vi "Voltage to temperature.vi"(8 "error in (no error)":errorcluster, 11 "Input Voltage (V)":dbl) -> (0 "error out":errorcluster, 3 "Temperature (C)":dbl)   [LabVIEW 2014]
doc: "Converts the input voltage to illuminance result."
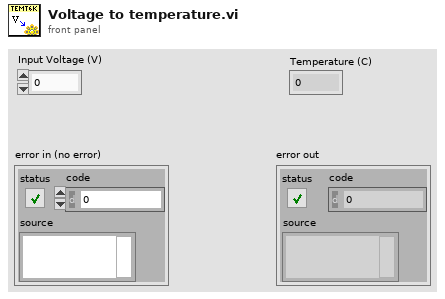
[diagram p1: front panel]
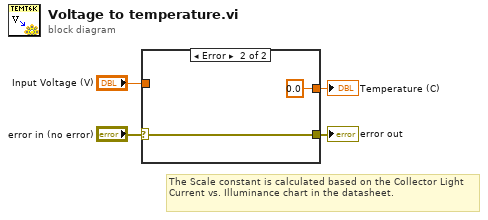
[diagram p0: block diagram]
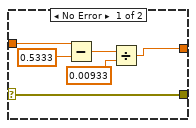
[diagram p2: hidden frame]
diagram:
  # "The Scale constant is calculated based on the Collector Light Current vs. Illuminance chart in the datasheet."
  n1 = case shown="Error" "error in (no error)" {
    selector: "error in (no error)" -> [w10 w12]
    tunnel: "Input Voltage (V)" -> [w9 _]
    tunnel: [w5 0.0] -> w3
    tunnel: [w10 w12] -> w1
    frame No Error {
      n2 = Subtract(x=w9, y=0.5333) -> (x-y=w7:dbl)
      n3 = Divide(x=w7, y=0.00933) -> (x/y=w5:dbl)
    }
    frame Error {
    }
  }
  "error out" <- w1
  "Temperature (C)" <- w3
